vi "ExampleAll.vi"() -> ()   [LabVIEW 2009]
uses:
  C/Program Files (x86)/National Instruments/LabVIEW 2018/user.lib/ATSpectrograph/ATSpectrograph.llb/atspectrograph_portPosition_typedef.ctl
  C/Program Files (x86)/National Instruments/LabVIEW 2018/user.lib/ATSpectrograph/ATSpectrograph.llb/atspectrograph_flipper_typedef.ctl
  C/Program Files (x86)/National Instruments/LabVIEW 2018/user.lib/ATSpectrograph/ATSpectrograph.llb/atspectrograph_slitIndex_typedef.ctl
  C/Program Files (x86)/National Instruments/LabVIEW 2018/user.lib/ATSpectrograph/ATSpectrograph.llb/atspectrograph_shutterMode_typedef.ctl
panel:
  in  "Device":i32 min=0 max=1
  in  "Tab Control":T1(tab)
  in  "Grating Offset":i32
  out "SetGratingOffset":string
  in  "Detector Offset":i32
  out "SetDetectorOffset":string
  out "WavelengthReset":string
  out "SetGrating":string
  in  "Grating":i32
  in  "Turret":i32
  out "SetTurret":string
  in  "SetGratingOffset":bool
  in  "SetDetectorOffset":bool
  in  "WavelengthReset":bool
  in  "SetGrating":bool
  in  "SetTurret":bool
  out "blaze":string
  out "Grating Offset":i32
  out "Detector Offset":i32
  out "offset":i32
  out "home":i32
  out "lines/mm":sgl format="%.2f"
  out "Grating":i32
  out "No Gratings":i32
  out "Turret":i32
  out "Is Grating ?":string
  out "GetGratingOffset":string
  out "GetDetectorOffset":string
  out "GetGratingInfo":string
  out "GetGrating":string
  out "GetNumberGratings":string
  out "GetTurret":string
  out "GratingIsPresent":string
  in  "Exit Port":T2
  in  "Entrance Port":T2
  out "GetCalibration":string
  out "SetNumberPixels":string
  out "SetPixelWidth":string
  out "Max Dispersion":sgl
  out "Min Dispersion":sgl
  in  "Number Pixels":i32 caption="Numeric"
  in  "Pixel Width":sgl caption="Numeric" format="%_3g"
  out "GotoZeroOrder":string
  out "SetWavelength":string
  in  "Wavelength":sgl format="%.2f"
  in  "GoToZeroOrder":bool
  out "Max Wavelength":sgl format="%.2f"
  out "Min Wavelength":sgl format="%.2f"
  out "Is Wavelength ?":string
  out "WavelengthIsPresent":string
  out "GetWavelengthLimits":string
  out "At Zero Order ?":string
  out "AtZeroOrder":string
  out "Wavelength":sgl format="%.2f"
  in  "SetWavelength 2":bool
  out "GetWavelength":string
  out "GetPixelWidth":string
  out "GetPixelCalibrationCoefficients":string
  out "GetNumberPixels":string
  out "Pixel Width":sgl format="%.2f"
  out "Number Pixels":i32
  out "A":sgl format="%.2f"
  out "B":sgl format="%.2f"
  out "C":sgl format="%.2f"
  out "D":sgl format="%.2f"
  in  "Slit":T3
  in  "SetSlit":bool
  in  "ResetSlit":bool
  in  "Slit Width":sgl format="%.2f"
  out "SetSlit":string
  out "ResetSlit":string
  out "Is Slit present ?":string
  out "GetSlitWidth":string
  out "SlitIsPresent":string
  out "Slit width (mm)":sgl format="%.2f"
  out "GetSlitZeroPosition":string
  out "SetSlitZeroPosition":string
  in  "SlitZeroPosition":i32
  in  "SlitZeroPositionGet":bool
  in  "SlitZeroPositionSet":bool caption="SetSlitZeroPosition"
  out "x1":i32
  out "y1":i32
  out "x2":i32
  out "y2":i32
  out "GetSlitCoefficients":string
  out "Shutter":T4
  in  "Mode":T4
  in  "SetShutter":bool
  out "Is Mode Possible ?":string
  out "Is Shutter ?":string
  out "SetShutter":string
  out "IsModePossible":string
  out "GetShutter":string
  out "ShutterIsPresent":string
  out "Port":T2
  in  "Flipper Port":T2
  in  "Flipper Mirror":T5
  out "High":sgl format="%.2f"
  in  "FlipperReset":bool
  out "FlipperReset":string
  in  "SetPort":bool
  out "Low":sgl format="%.2f"
  out "Is Flipper ?":string
  out "SetPort":string
  out "GetCCDLimits":string
  out "FlipperIsPresent":string
  out "GetFlipperMirror":string
  out "SetFlipperMirrorPosition":string
  in  "SetFlipperMirrorPosition":bool
  in  "Position":i32
  out "GetFlipperMirrorPosition":string
  out "Mirror Max Position":i32
  out "Mirror Position":i32
  out "GetFlipperMirrorMaxPosition":string
  in  "ResetFocusMirror":bool
  in  "MoveFocusMirror":bool
  in  "Steps":i32
  out "FocusMirrorReset":string
  out "SetFocusMirror":string
  out "FocusMirrorIsPresent":string
  out "GetFocusMirror":string
  out "GetFocusMirrorMaxSteps":string
  out "Max Steps":i32
  out "Is Focus Mirror ?":string
  out "Focus":i32
  in  "Iris":T2
  in  "SetIris":bool
  out "SetIris":string
  in  "Value":i32
  out "Iris Value":i32
  out "Is Iris ?":string
  out "GetIris":string
  out "IrisIsPresent":string
  in  "Filter info":string caption="String"
  out "Filter Info":string
  in  "SetFilterInfo":bool
  out "SetFilterInfo":string
  in  "Filter":i32
  in  "SetFilter":bool
  out "Filter":i32
  out "Is Filter ?":string
  out "SetFilter":string
  out "GetFilterInfo":string
  out "GetFilter":string
  out "FilterIsPresent":string
  in  "ResetFilter 2":bool
  out "ResetFilter":string
  in  "Line":i32
  out "Line 2":i32
  in  "State":i32
  in  "Set Accessory":bool
  out "Line 1":i32
  out "Is Accessory ?":string
  out "SetAccessory":string
  out "GetAccessory":string
  out "AccessoryIsPresent":string
  in  "Set Params":bool
  out "Set Optical Parameters":string
  in  "Focal tilt":sgl format="%.2f"
  in  "Angular deviation":sgl format="%.2f"
  in  "Focal length":sgl format="%.4f"
  out "Initializing":bool
  in  "STOP if TRUE":bool
  out "Focal tilt":sgl format="%.2f"
  out "Angular deviation":sgl format="%.2f"
  out "Focal length":sgl format="%.4f"
  out "Serial Number":string
  out "No of devices":i32
  out "GetOpticalParameters":string
  out "GetSerialNumber":string
  out "GetNumberDevices":string
  out "Close":string
  out "Initialize":string
  # "INITIALIZATION"
  # "SDK RETURN VALUES"
  # "SHAMROCK PARAMETERS"
  # "ACTIONS"
  # "SDK RETURN VALUES"
  # "SHAMROCK PARAMETERS"
  # "ACTIONS"
  # "SDK RETURN VALUES"
  # "SHAMROCK PARAMETERS"
  # "ACTIONS"
  # "nm"
  # "Dispersion range"
  # "SDK RETURN VALUES"
  # "SHAMROCK PARAMETERS"
  # "ACTIONS"
  # "Slit Zero Position"
  # "SDK RETURN VALUES"
  # "SHAMROCK PARAMETERS"
  # "ACTIONS"
  # "SDK RETURN VALUES"
  # "SHAMROCK PARAMETERS"
  # "ACTIONS"
  # "SDK RETURN VALUES"
  # "SHAMROCK PARAMETERS"
  # "ACTIONS"
  # "SDK RETURN VALUES"
  # "SHAMROCK PARAMETERS"
  # "ACTIONS"
  # "SDK RETURN VALUES"
  # "SHAMROCK PARAMETERS"
  # "ACTIONS"
  # "SDK RETURN VALUES"
  # "SHAMROCK PARAMETERS"
  # "ACTIONS"
  # "line"
  # "to state"
  # "SDK RETURN VALUES"
  # "SHAMROCK PARAMETERS"
  # "ACTIONS"
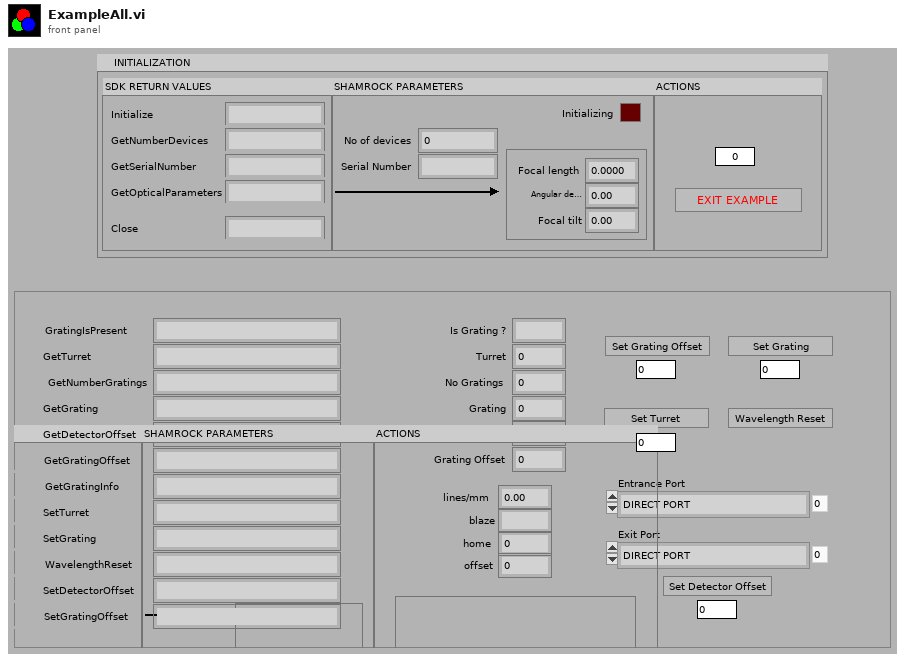
[diagram p1: front panel]
types:
  T1 = enum32{"GRATINGS", "WAVELENGTH", "SLIT", "SHUTTER", "FLIPPER MIRROR", "FOCUS MIRROR", "IRIS", "FILTER", "ACCESSORY", "OPTICALPARAMS"}
  T2 = typedef "atspectrograph_portPosition_typedef.ctl" = enum32{"DIRECT PORT", "SIDE PORT"}
  T3 = typedef "atspectrograph_slitIndex_typedef.ctl" = enum32{"Reserved (0)", "INPUT SIDE", "INPUT DIRECT", "OUTPUT SIDE", "OUTPUT DIRECT"}
  T4 = typedef "atspectrograph_shutterMode_typedef.ctl" = enum32{"CLOSED", "OPEN", "BNC"}
  T5 = typedef "atspectrograph_flipper_typedef.ctl" = enum32{"Reserved (0)", "INPUT FLIPPER", "OUTPUT FLIPPER"}
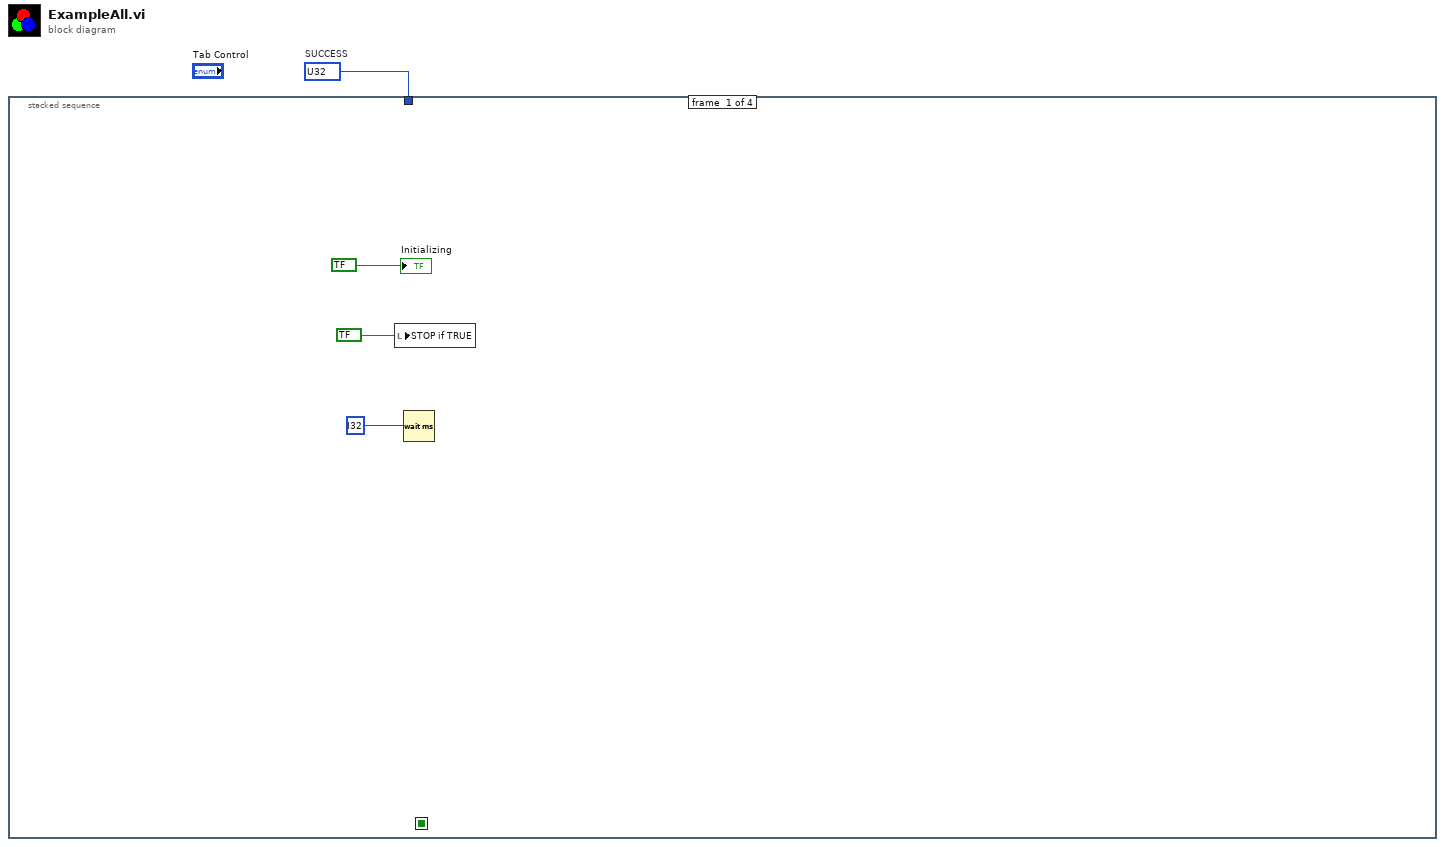
[diagram p0: block diagram]
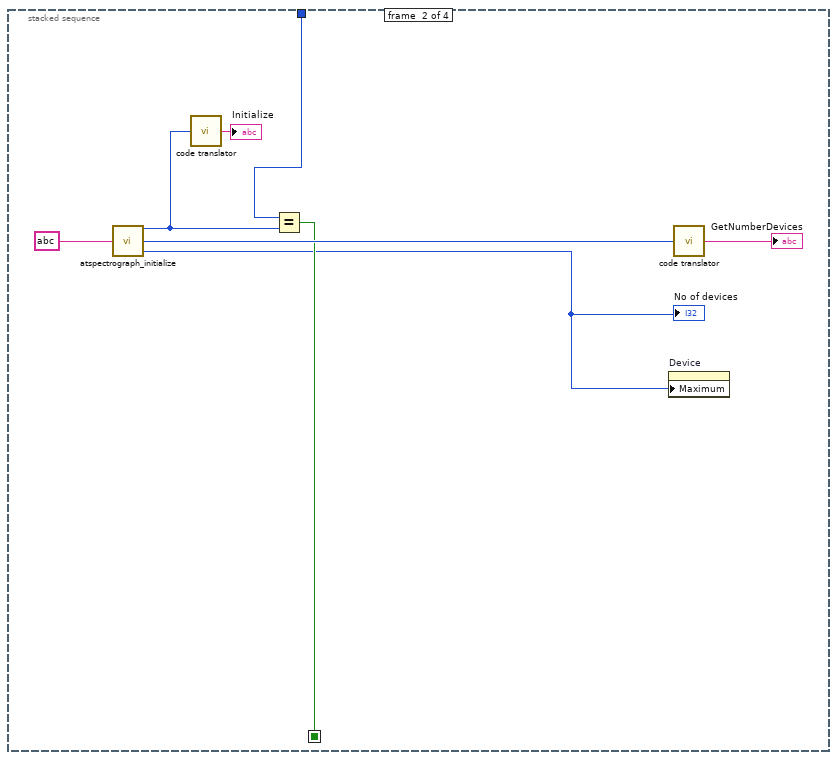
[diagram p2: hidden frame]
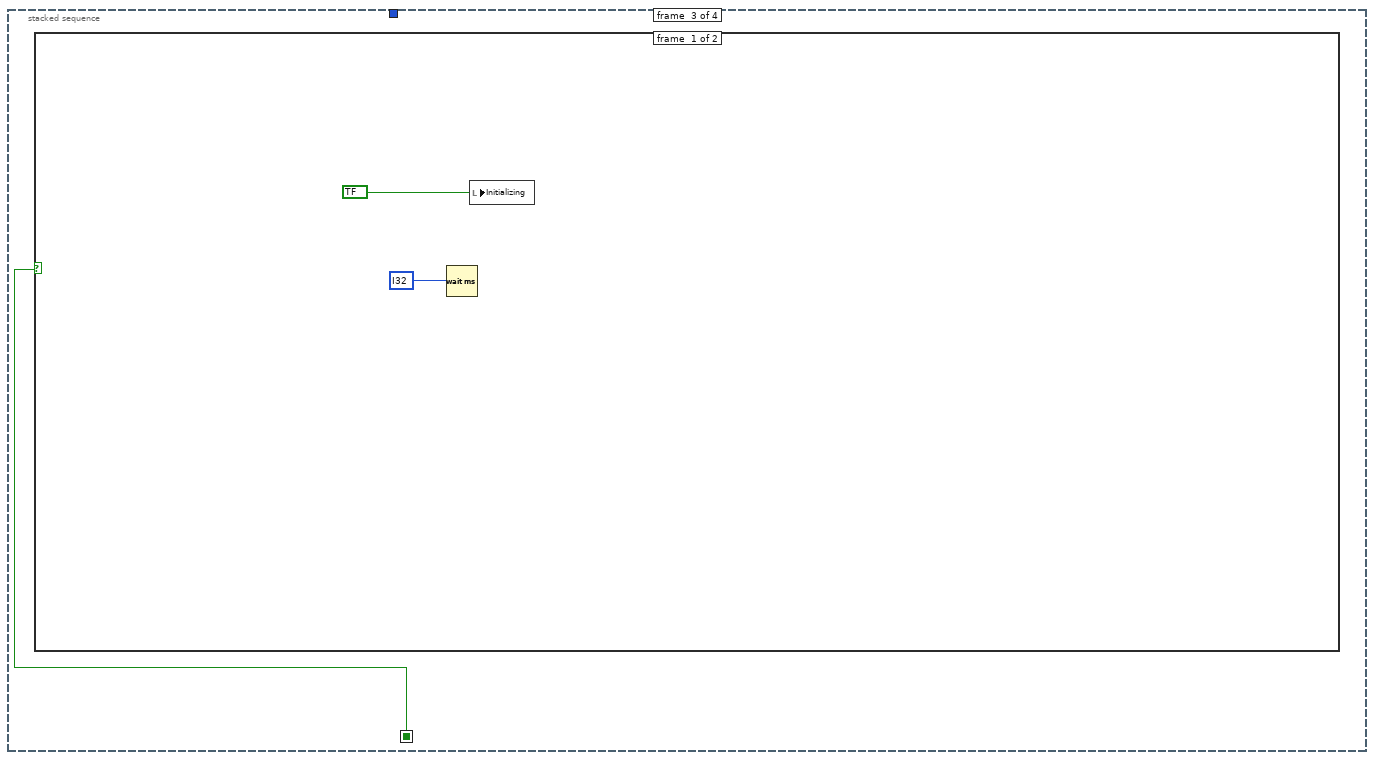
[diagram p3: hidden frame]
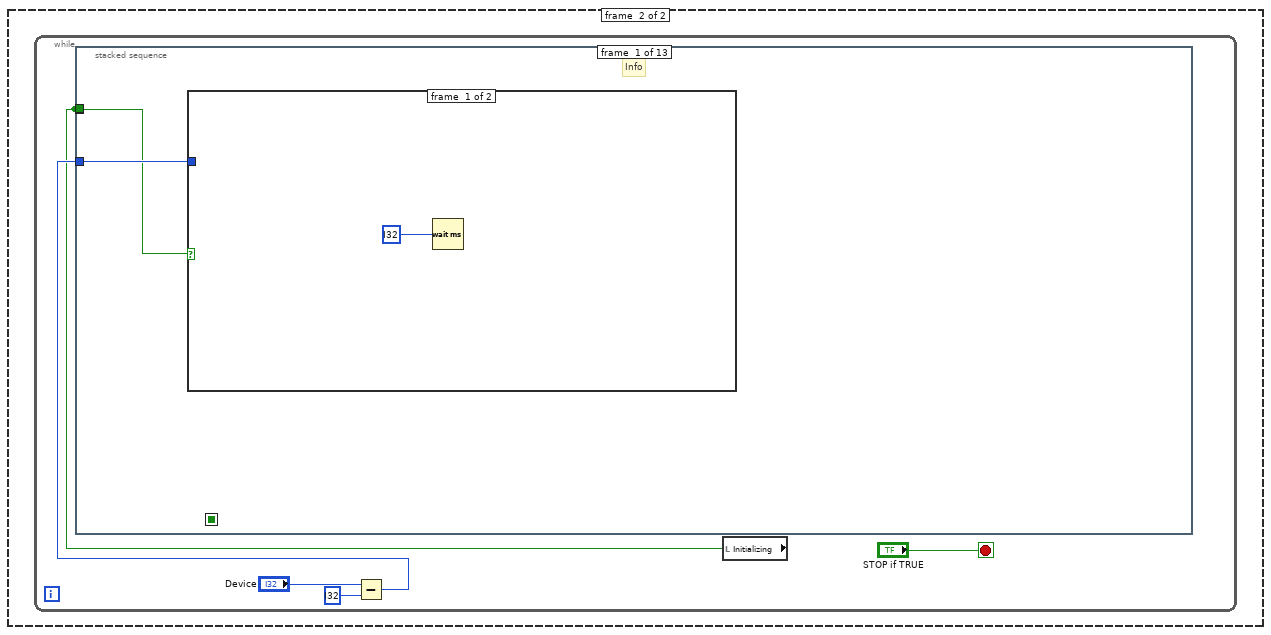
[diagram p4: hidden frame]
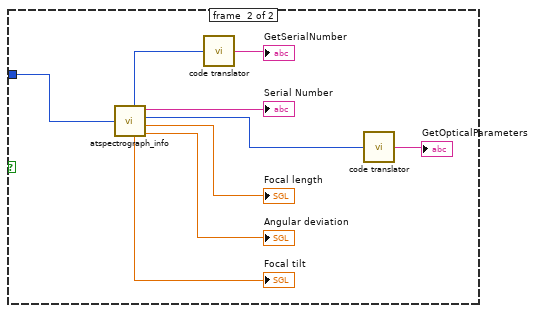
[diagram p5: hidden frame]
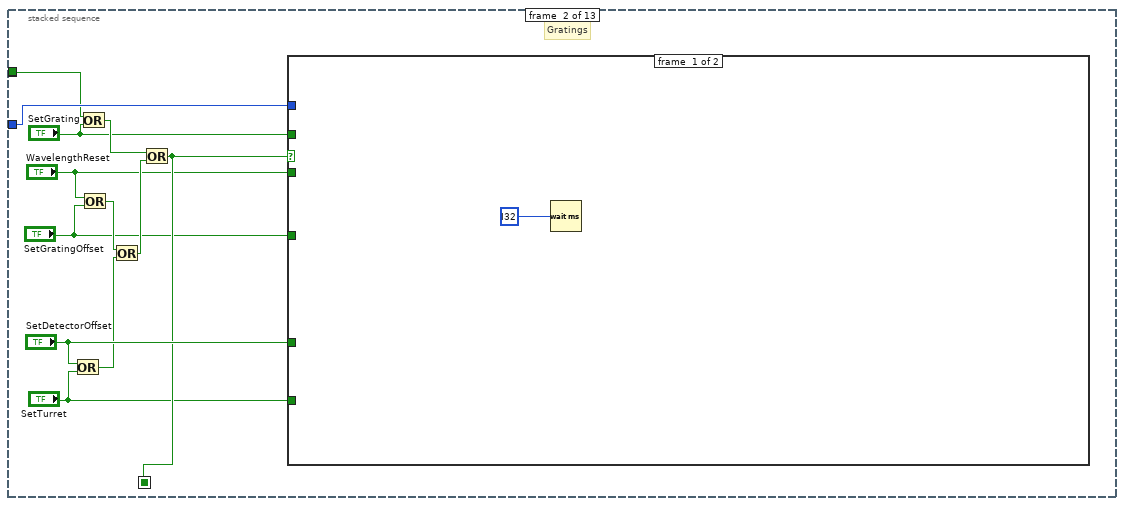
[diagram p6: hidden frame]
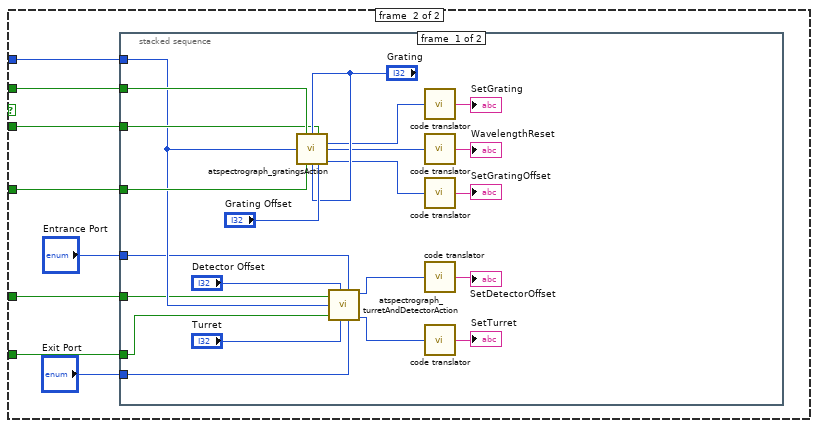
[diagram p7: hidden frame]
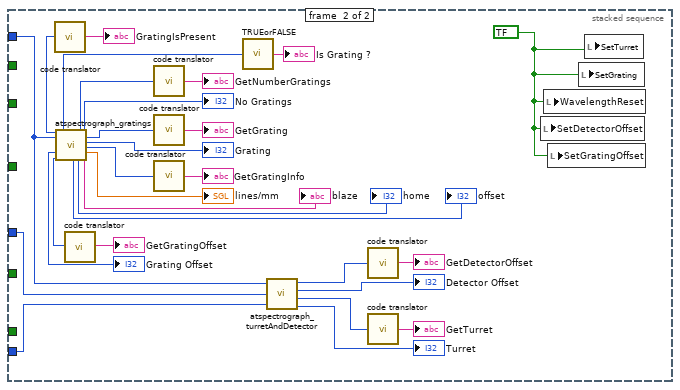
[diagram p8: hidden frame]
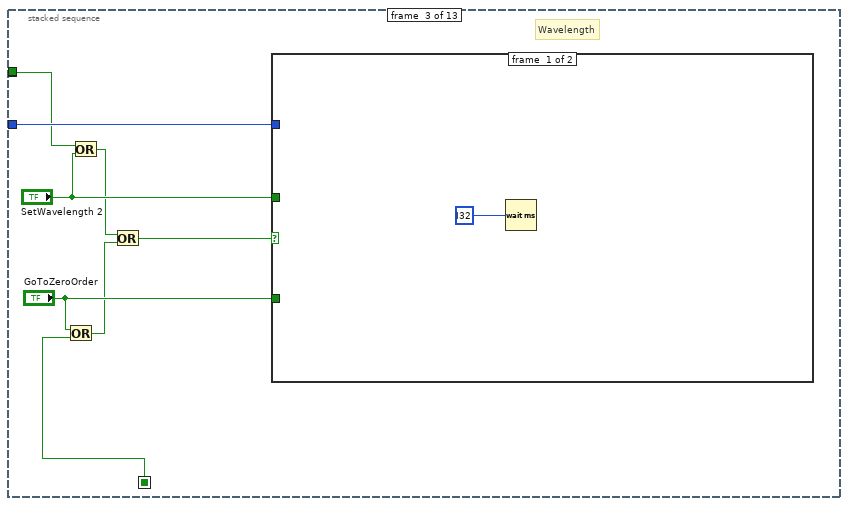
[diagram p9: hidden frame]
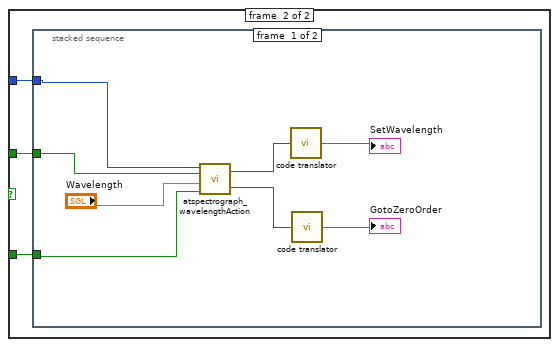
[diagram p10: hidden frame]
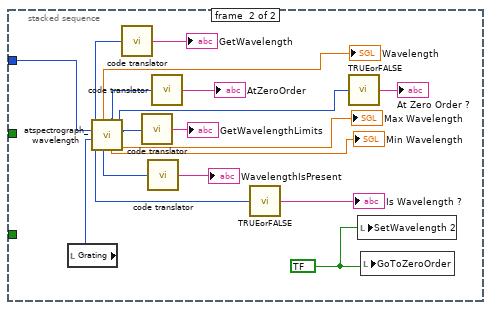
[diagram p11: hidden frame]
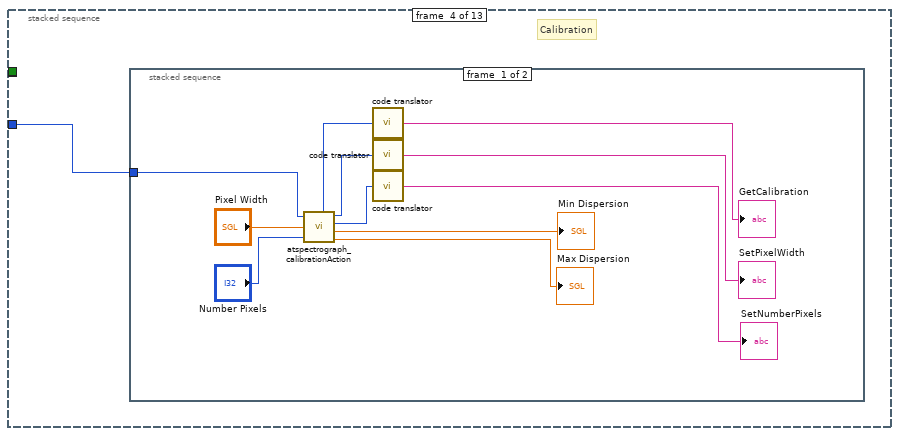
[diagram p12: hidden frame]
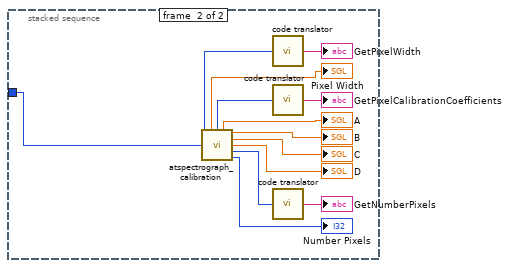
[diagram p13: hidden frame]
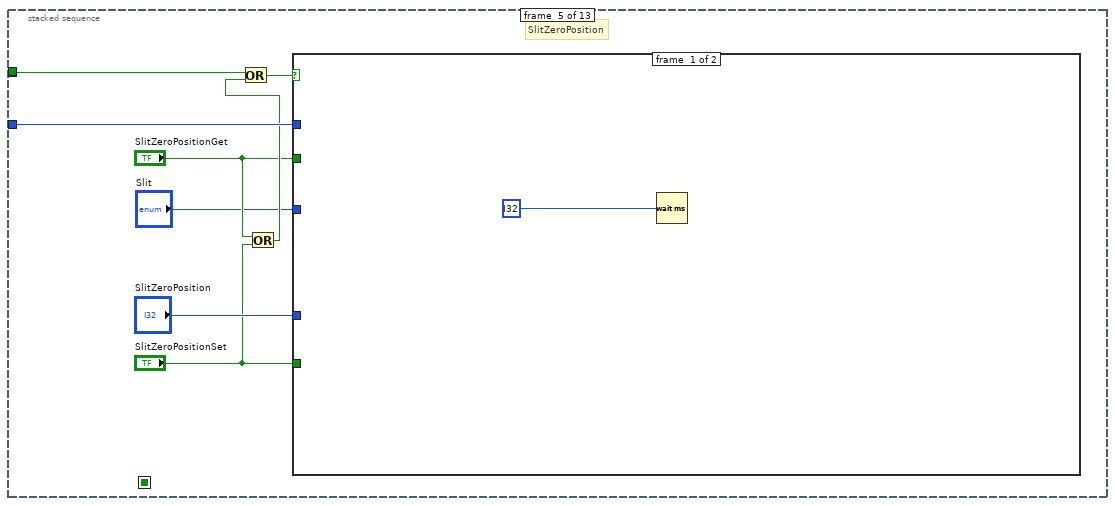
[diagram p14: hidden frame]
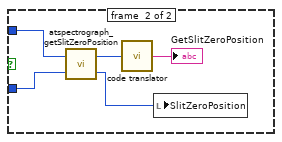
[diagram p16: hidden frame]
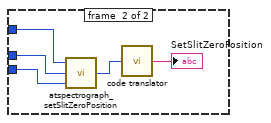
[diagram p17: hidden frame]
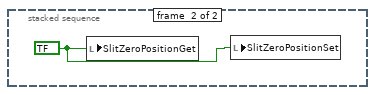
[diagram p18: hidden frame]
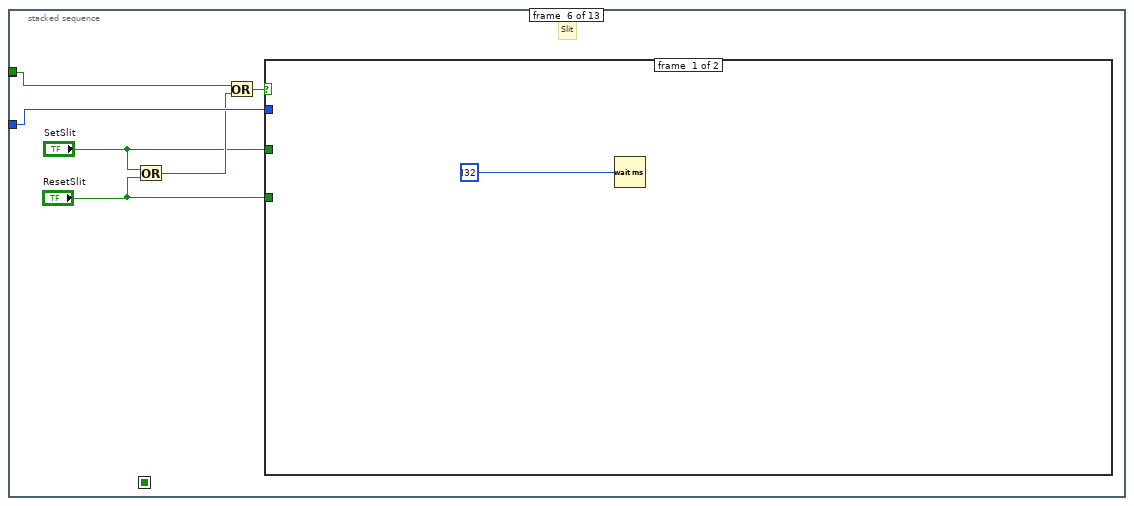
[diagram p19: hidden frame]
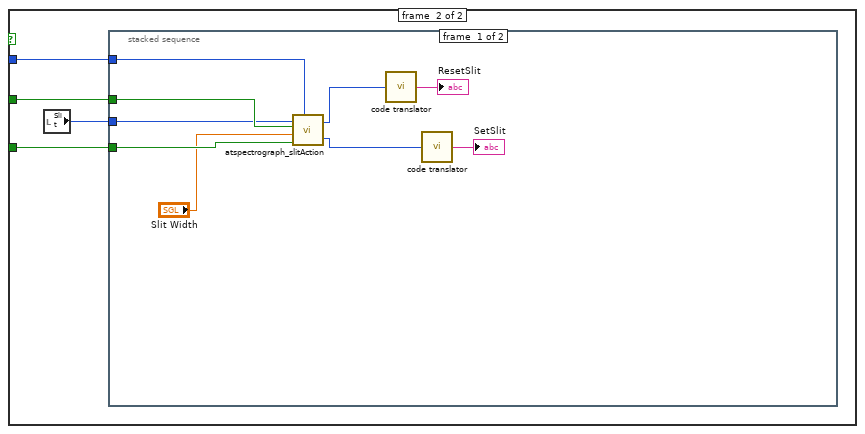
[diagram p20: hidden frame]
diagram:
  w1 = u32 ?  # SUCCESS
  n1 = stacked-sequence {
    seq-local: [_ w6 _ _] -> [_ _ w13 _]
    tunnel: w1 -> [_ w12 _ _]
    frame #0 {
      n2 = local write "STOP if TRUE"(bool ?) -> ()
      n3 = Wait (ms)(milliseconds to wait=i32 ?) -> ()  [unwired: 1 out]
      "Initializing" <- bool ?
    }
    frame #1 {
      n4 = call "atspectrograph_initialize.vi"("Initialization path"=string ?) -> ("RC_Initialize"=w9:u32, "RC_GetNumberDevices"=w8:u32, "No Devices"=w5:i32)
      "No of devices" <- w5
      n5 = call "code translator.vi"("Error code"=w9) -> ("Error description"=→"Initialize":string)
      n6 = Equal?(x=w12, y=w9) -> (x = y?=w6:bool)
      n7 = property on="Device" class="DigNum (strict)"("Maximum"=w5) -> ()  [unwired: 2 in, 2 out]
      n8 = call "code translator.vi"("Error code"=w8) -> ("Error description"=→"GetNumberDevices":string)
    }
    frame #2 {
      n9 = case shown="True" w13 {
        frame #0 {
          n10 = Wait (ms)(milliseconds to wait=i32 ?) -> ()  [unwired: 1 out]
          n11 = local write "Initializing"(bool ?) -> ()
        }
        frame #1 {
          n12 = while {
            stop <- "STOP if TRUE" stop-if-true
            n13 = Subtract(x="Device", y=i32 ?) -> (x-y=w19:i32)
            n14 = local read "Initializing"() -> (w16:bool)
            n15 = stacked-sequence {
              seq-local: [_ w37 _ _ _ _ _ _ _ _ _ _ _] -> [_ _ w111 _ _ _ _ _ _ _ _ _ _]
              tunnel: w19 -> [w22 w44 w112 w143 w175 w201 w237 w267 w312 w340 w368 w401 w425]
              tunnel: w16 -> [w21 w40 w108 _ w173 w203 w234 w262 w311 w339 w364 w398 _]
              tunnel: w16 -> [_ _ _ _ _ _ _ _ _ _ _ _ _]
              frame #0 {
                # "Info"
                n16 = case shown="True" w21 {
                  tunnel: w22 -> [_ w24]
                  frame #0 {
                    n17 = Wait (ms)(milliseconds to wait=i32 ?) -> ()  [unwired: 1 out]
                  }
                  frame #1 {
                    n18 = call "atspectrograph_info.vi"("Device No"=w24) -> ("RC_GetSerialNumber"=w28:u32, "Focal Tilt"=→"Focal tilt":sgl, "Serial Number"=→"Serial Number":string, "RC_GetOpticalParameters"=w26:u32, "Focal Length"=→"Focal length":sgl, "Angular Deviation"=→"Angular deviation":sgl)
                    n19 = call "code translator.vi"("Error code"=w28) -> ("Error description"=→"GetSerialNumber":string)
                    n20 = call "code translator.vi"("Error code"=w26) -> ("Error description"=→"GetOpticalParameters":string)
                  }
                }
              }
              frame #1 {
                # "Gratings"
                n21 = Or(x="SetDetectorOffset", y="SetTurret") -> (x .or. y?=w41:bool)
                n22 = Or(x=w40, y="SetGrating") -> (x .or. y?=w39:bool)
                n23 = Or(x="WavelengthReset", y="SetGratingOffset") -> (x .or. y?=w42:bool)
                n24 = Or(x=w42, y=w41) -> (x .or. y?=w38:bool)
                n25 = Or(x=w39, y=w38) -> (x .or. y?=w37:bool)
                n26 = case shown="True" w37 {
                  tunnel: w44 -> [_ w53]
                  tunnel: "SetDetectorOffset" -> [_ w52]
                  tunnel: "SetTurret" -> [_ w51]
                  tunnel: "WavelengthReset" -> [_ w50]
                  tunnel: "SetGratingOffset" -> [_ w49]
                  tunnel: "SetGrating" -> [_ w48]
                  frame #0 {
                    n27 = Wait (ms)(milliseconds to wait=i32 ?) -> ()  [unwired: 1 out]
                  }
                  frame #1 {
                    n28 = stacked-sequence {
                      tunnel: w48 -> [w65 _]
                      tunnel: w53 -> [w62 w78]
                      tunnel: w50 -> [w64 _]
                      tunnel: w49 -> [w63 _]
                      tunnel: w52 -> [w58 _]
                      tunnel: w51 -> [w59 _]
                      tunnel: "Entrance Port" -> [w55 w77]
                      tunnel: "Exit Port" -> [w54 w76]
                      frame #0 {
                        n29 = call "atspectrograph_gratingsAction.vi"("WavelengthReset"=w64, "Grating Offset"="Grating Offset", 7:"Grating"="Grating", 8:"Grating"="Grating", "SetGrating"=w65, "SetGratingOffset"=w63, "Device No"=w62) -> ("RC_SetGrating"=w72:u32, "RC_WavelengthReset"=w69:u32, "RC_SetGratingOffset"=w67:u32)  [unwired: 6 in]
                        n30 = call "atspectrograph_turretAndDetectorAction.vi"("SetDetectorOffset"=w58, "Detector Offset"="Detector Offset", "Device No"=w62, "SetTurret"=w59, "Turret"="Turret", "Entrance Port"=w55, "Exit Port"=w54) -> ("RC_SetDetectorOffset"=w57:u32, "RC_SetTurret"=w56:u32)  [unwired: 2 in]
                        n31 = call "code translator.vi"("Error code"=w72) -> ("Error description"=→"SetGrating":string)
                        n32 = call "code translator.vi"("Error code"=w69) -> ("Error description"=→"WavelengthReset":string)
                        n33 = call "code translator.vi"("Error code"=w67) -> ("Error description"=→"SetGratingOffset":string)
                        n34 = call "code translator.vi"("Error code"=w57) -> ("Error description"=→"SetDetectorOffset":string)
                        n35 = call "code translator.vi"("Error code"=w56) -> ("Error description"=→"SetTurret":string)
                      }
                      frame #1 {
                        w104 = bool ?
                        n36 = call "atspectrograph_gratings.vi"("Device No"=w78) -> ("No Gratings"=→"No Gratings":i32, "RC_GetNumberGratings"=w93:u32, "Is Present"=w84:i32, "RC_GratingIsPresent"=w96:u32, "RC_GetGrating"=w91:u32, "Grating"=→"Grating":i32, "RC_GetGratingInfo"=w89:u32, "Lines/mm"=→"lines/mm":sgl, "Grating Offset"=→"Grating Offset":i32, "Blaze"=→"blaze":string, "Home"=→"home":i32, "Offset"=→"offset":i32, "RC_GetGratingOffset"=w86:u32)  [unwired: 6 in]
                        n37 = call "code translator.vi"("Error code"=w96) -> ("Error description"=→"GratingIsPresent":string)
                        n38 = call "code translator.vi"("Error code"=w86) -> ("Error description"=→"GetGratingOffset":string)
                        n39 = call "code translator.vi"("Error code"=w93) -> ("Error description"=→"GetNumberGratings":string)
                        n40 = call "code translator.vi"("Error code"=w91) -> ("Error description"=→"GetGrating":string)
                        n41 = call "code translator.vi"("Error code"=w89) -> ("Error description"=→"GetGratingInfo":string)
                        n42 = call "TRUEorFALSE.vi"("bool number"=w84) -> ("String"=→"Is Grating ?":string)
                        n43 = call "atspectrograph_turretAndDetector.vi"("Device No"=w78, "Entrance Port"=w77, "Exit Port"=w76) -> ("RC_GetDetectorOffset"=w82:u32, "Detector Offset"=→"Detector Offset":i32, "RC_GetTurret"=w80:u32, "Turret"=→"Turret":i32)
                        n44 = call "code translator.vi"("Error code"=w82) -> ("Error description"=→"GetDetectorOffset":string)
                        n45 = call "code translator.vi"("Error code"=w80) -> ("Error description"=→"GetTurret":string)
                        n46 = local write "SetDetectorOffset"(w104) -> ()
                        n47 = local write "WavelengthReset"(w104) -> ()
                        n48 = local write "SetGratingOffset"(w104) -> ()
                        n49 = local write "SetGrating"(w104) -> ()
                        n50 = local write "SetTurret"(w104) -> ()
                      }
                    }
                  }
                }
              }
              frame #2 {
                # "Wavelength"
                n51 = Or(x="GoToZeroOrder", y=w111) -> (x .or. y?=w106:bool)
                n52 = Or(x=w108, y="SetWavelength 2") -> (x .or. y?=w107:bool)
                n53 = Or(x=w107, y=w106) -> (x .or. y?=w105:bool)
                n54 = case shown="True" w105 {
                  tunnel: "SetWavelength 2" -> [_ w116]
                  tunnel: "GoToZeroOrder" -> [_ w115]
                  tunnel: w112 -> [_ w114]
                  frame #0 {
                    n55 = Wait (ms)(milliseconds to wait=i32 ?) -> ()  [unwired: 1 out]
                  }
                  frame #1 {
                    n56 = stacked-sequence {
                      tunnel: w116 -> [w122 _]
                      tunnel: w115 -> [w123 _]
                      tunnel: w114 -> [w121 w137]
                      frame #0 {
                        n57 = call "atspectrograph_wavelengthAction.vi"("GoToZeroOrder"=w123, "Wavelength"="Wavelength", "SetWavelength"=w122, "Device No"=w121) -> ("RC_GotoZeroOrder"=w118:u32, "RC_SetWavelength"=w120:u32)
                        n58 = call "code translator.vi"("Error code"=w120) -> ("Error description"=→"SetWavelength":string)
                        n59 = call "code translator.vi"("Error code"=w118) -> ("Error description"=→"GotoZeroOrder":string)
                      }
                      frame #1 {
                        w142 = bool ?
                        n60 = local read "Grating"() -> (w138:i32)
                        n61 = call "atspectrograph_wavelength.vi"("Grating No"=w138, "Device No"=w137) -> ("Is Present"=w126:i32, "RC_WavelengthIsPresent"=w130:u32, "Min Wavelength"=→"Min Wavelength":sgl, "Max Wavelength"=→"Max Wavelength":sgl, "RC_GetWavelengthLimits"=w132:u32, "RC_GetWavelength"=w136:u32, "Wavelength"=→"Wavelength":sgl, "RC_AtZeroOrder"=w134:u32, "At Zero Order"=w128:i32)
                        n62 = call "code translator.vi"("Error code"=w136) -> ("Error description"=→"GetWavelength":string)
                        n63 = call "code translator.vi"("Error code"=w132) -> ("Error description"=→"GetWavelengthLimits":string)
                        n64 = call "code translator.vi"("Error code"=w130) -> ("Error description"=→"WavelengthIsPresent":string)
                        n65 = call "code translator.vi"("Error code"=w134) -> ("Error description"=→"AtZeroOrder":string)
                        n66 = call "TRUEorFALSE.vi"("bool number"=w126) -> ("String"=→"Is Wavelength ?":string)
                        n67 = call "TRUEorFALSE.vi"("bool number"=w128) -> ("String"=→"At Zero Order ?":string)
                        n68 = local write "SetWavelength 2"(w142) -> ()
                        n69 = local write "GoToZeroOrder"(w142) -> ()
                      }
                    }
                  }
                }
              }
              frame #3 {
                # "Calibration"
                n70 = stacked-sequence {
                  tunnel: w143 -> [w145 w164]
                  frame #0 {
                    n71 = call "atspectrograph_calibrationAction.vi"("Device No"=w145, "Set Pixel Width"="Pixel Width", "Set Number Pixels"="Number Pixels") -> ("RC_SetPixelWidth"=w152:u32, "RC_SetNumberPixels"=w150:u32, "Wavelength First Pixel"=→"Min Dispersion":sgl, "Wavelength Last Pixel"=→"Max Dispersion":sgl, "RC_GetCalibration"=w154:u32)
                    n72 = call "code translator.vi"("Error code"=w154) -> ("Error description"=→"GetCalibration":string)
                    n73 = call "code translator.vi"("Error code"=w152) -> ("Error description"=→"SetPixelWidth":string)
                    n74 = call "code translator.vi"("Error code"=w150) -> ("Error description"=→"SetNumberPixels":string)
                  }
                  frame #1 {
                    n75 = call "atspectrograph_calibration.vi"("Device No"=w164) -> ("B"=→"B":sgl, "C"=→"C":sgl, "D"=→"D":sgl, "RC_GetNumberPixels"=w156:u32, "Number Pixels"=→"Number Pixels":i32, "A"=→"A":sgl, "RC_GetPixelCalibrationCoefficients"=w161:u32, "Width"=→"Pixel Width":sgl, "RC_GetPixelWidth"=w163:u32)  [unwired: 2 in, 4 out]
                    n76 = call "code translator.vi"("Error code"=w163) -> ("Error description"=→"GetPixelWidth":string)
                    n77 = call "code translator.vi"("Error code"=w161) -> ("Error description"=→"GetPixelCalibrationCoefficients":string)
                    n78 = call "code translator.vi"("Error code"=w156) -> ("Error description"=→"GetNumberPixels":string)
                  }
                }
              }
              frame #4 {
                # "SlitZeroPosition"
                n79 = Or(x="SlitZeroPositionGet", y="SlitZeroPositionSet") -> (x .or. y?=w170:bool)
                n80 = Or(x=w173, y=w170) -> (x .or. y?=w174:bool)
                n81 = case shown="True" w174 {
                  tunnel: w175 -> [_ w181]
                  tunnel: "SlitZeroPositionGet" -> [_ w180]
                  tunnel: "SlitZeroPositionSet" -> [_ w179]
                  tunnel: "Slit" -> [_ w178]
                  tunnel: "SlitZeroPosition" -> [_ w177]
                  frame #0 {
                    n82 = Wait (ms)(milliseconds to wait=i32 ?) -> ()  [unwired: 1 out]
                  }
                  frame #1 {
                    n83 = stacked-sequence {
                      tunnel: w181 -> [w185 _]
                      tunnel: w180 -> [w186 _]
                      tunnel: w179 -> [w184 _]
                      tunnel: w178 -> [w183 _]
                      tunnel: w177 -> [w182 _]
                      frame #0 {
                        n84 = case shown="True" w186 {
                          tunnel: w185 -> [_ w191]
                          tunnel: w183 -> [_ w187]
                          frame #0 {
                          }
                          frame #1 {
                            n85 = call "atspectrograph_getSlitZeroPosition.vi"("Slit Index"=w187, "Device No"=w191) -> ("Slit Zero Position (mm)"=w188:i32, "RC_GetSlitZeroPosition"=w190:u32)
                            n86 = call "code translator.vi"("Error code"=w190) -> ("Error description"=→"GetSlitZeroPosition":string)
                            n87 = local write "SlitZeroPosition"(w188) -> ()
                          }
                        }
                        n88 = case shown="True" w184 {
                          tunnel: w185 -> [_ w196]
                          tunnel: w183 -> [_ w193]
                          tunnel: w182 -> [_ w192]
                          frame #0 {
                          }
                          frame #1 {
                            n89 = call "atspectrograph_setSlitZeroPosition.vi"("Offset"=w192, "Slit Index"=w193, "Device No"=w196) -> ("RC_SetSlitZeroPosition"=w195:u32)
                            n90 = call "code translator.vi"("Error code"=w195) -> ("Error description"=→"SetSlitZeroPosition":string)
                          }
                        }
                      }
                      frame #1 {
                        w197 = bool ?
                        n91 = local write "SlitZeroPositionGet"(w197) -> ()
                        n92 = local write "SlitZeroPositionSet"(w197) -> ()
                      }
                    }
                  }
                }
              }
              frame #5 {
                # "Slit"
                n93 = Or(x="SetSlit", y="ResetSlit") -> (x .or. y?=w200:bool)
                n94 = Or(x=w203, y=w200) -> (x .or. y?=w202:bool)
                n95 = case shown="True" w202 {
                  tunnel: w201 -> [_ w208]
                  tunnel: "SetSlit" -> [_ w207]
                  tunnel: "ResetSlit" -> [_ w206]
                  frame #0 {
                    n96 = Wait (ms)(milliseconds to wait=i32 ?) -> ()  [unwired: 1 out]
                  }
                  frame #1 {
                    n97 = local read "Slit"() -> (w205:T3)
                    n98 = stacked-sequence {
                      tunnel: w208 -> [w217 w225]
                      tunnel: w207 -> [w216 _]
                      tunnel: w206 -> [w215 _]
                      tunnel: w205 -> [w214 w233]
                      frame #0 {
                        n99 = call "atspectrograph_slitAction.vi"("Slit"=w214, "Set Slit"=w216, "Slit Width"="Slit Width", "Reset Slit"=w215, "Device No"=w217) -> ("RC_ResetSlit"=w209:u32, "RC_SetSlit"=w211:u32)
                        n100 = call "code translator.vi"("Error code"=w209) -> ("Error description"=→"ResetSlit":string)
                        n101 = call "code translator.vi"("Error code"=w211) -> ("Error description"=→"SetSlit":string)
                      }
                      frame #1 {
                        w218 = bool ?
                        n102 = call "atspectrograph_slit.vi"("Device No"=w225, "Slit Index"=w233) -> ("RC_SlitIsPresent"=w226:u32, "RC_GetSlitWidth"=w227:u32, "Is Present"=w228:i32, "Slit Width (mm)"=→"Slit width (mm)":sgl)
                        n103 = call "atspectrograph_getSlitCoefficients.vi"("Device No"=w225) -> ("y2"=→"y2":i32, "x2"=→"x2":i32, "y1"=→"y1":i32, "x1"=→"x1":i32, "RC_GetSlitCoefficients"=w223:u32)
                        n104 = call "code translator.vi"("Error code"=w226) -> ("Error description"=→"SlitIsPresent":string)
                        n105 = call "code translator.vi"("Error code"=w227) -> ("Error description"=→"GetSlitWidth":string)
                        n106 = call "TRUEorFALSE.vi"("bool number"=w228) -> ("String"=→"Is Slit present ?":string)
                        n107 = call "code translator.vi"("Error code"=w223) -> ("Error description"=→"GetSlitCoefficients":string)
                        n108 = local write "ResetSlit"(w218) -> ()
                        n109 = local write "SetSlit"(w218) -> ()
                      }
                    }
                  }
                }
              }
              frame #6 {
                # "Shutter"
                n110 = Or(x=w234, y="SetShutter") -> (x .or. y?=w235:bool)
                n111 = case shown="True" w235 {
                  tunnel: w237 -> [_ w240]
                  tunnel: "SetShutter" -> [_ w239]
                  frame #0 {
                    n112 = Wait (ms)(milliseconds to wait=i32 ?) -> ()  [unwired: 1 out]
                  }
                  frame #1 {
                    n113 = stacked-sequence {
                      seq-local: ["Mode" _] -> [_ w257]
                      tunnel: w240 -> [w244 w258]
                      tunnel: w239 -> [w245 _]
                      frame #0 {
                        n114 = call "atspectrograph_shutterAction.vi"("Mode"="Mode", "SetShutter"=w245, "Device No"=w244) -> ("RC_SetShutter"=w243:u32)
                        n115 = call "code translator.vi"("Error code"=w243) -> ("Error description"=→"SetShutter":string)
                      }
                      frame #1 {
                        n116 = call "atspectrograph_shutter.vi"("Device No"=w258, "Mode"=w257) -> ("RC_ShutterIsPresent"=w256:u32, "Is Mode Possible"=w248:i32, "Is Present"=w249:i32, "RC_GetShutter"=w254:u32, "Shutter"=→"Shutter":T4, "RC_IsModePossible"=w252:u32)
                        n117 = call "code translator.vi"("Error code"=w256) -> ("Error description"=→"ShutterIsPresent":string)
                        n118 = call "code translator.vi"("Error code"=w252) -> ("Error description"=→"IsModePossible":string)
                        n119 = call "code translator.vi"("Error code"=w254) -> ("Error description"=→"GetShutter":string)
                        n120 = call "TRUEorFALSE.vi"("bool number"=w248) -> ("String"=→"Is Mode Possible ?":string)
                        n121 = call "TRUEorFALSE.vi"("bool number"=w249) -> ("String"=→"Is Shutter ?":string)
                        n122 = local write "SetShutter"(bool ?) -> ()
                      }
                    }
                  }
                }
              }
              frame #7 {
                # "Flipper Mirror"
                n123 = Or(x=w262, y="SetFlipperMirrorPosition") -> (x .or. y?=w261:bool)
                n124 = Or(x="SetPort", y="FlipperReset") -> (x .or. y?=w264:bool)
                n125 = Or(x=w261, y=w264) -> (x .or. y?=w263:bool)
                n126 = case shown="True" w263 {
                  tunnel: "SetPort" -> [_ w273]
                  tunnel: "FlipperReset" -> [_ w272]
                  tunnel: w267 -> [_ w271]
                  tunnel: "SetFlipperMirrorPosition" -> [_ w269]
                  frame #0 {
                    n127 = Wait (ms)(milliseconds to wait=i32 ?) -> ()  [unwired: 1 out]
                  }
                  frame #1 {
                    n128 = stacked-sequence {
                      tunnel: w273 -> [w282 _]
                      tunnel: w272 -> [w281 _]
                      tunnel: w271 -> [w284 w294]
                      tunnel: "Flipper Mirror" -> [w283 w295]
                      tunnel: w269 -> [w278 _]
                      frame #0 {
                        n129 = call "atspectrograph_flipperMirrorAction.vi"("Device No"=w284, "Position"="Position", "SetFlipperMirrorPosition"=w278, "FlipperReset"=w281, 8:"Flipper Port", "SetPort"=w282, 10:w283) -> ("RC_SetFlipperMirrorPosition"=w276:u32, "RC_FlipperReset"=w280:u32, "RC_SetPort"=w279:u32)  [unwired: 1 in]
                        n130 = call "code translator.vi"("Error code"=w279) -> ("Error description"=→"SetPort":string)
                        n131 = call "code translator.vi"("Error code"=w280) -> ("Error description"=→"FlipperReset":string)
                        n132 = call "code translator.vi"("Error code"=w276) -> ("Error description"=→"SetFlipperMirrorPosition":string)
                      }
                      frame #1 {
                        w296 = bool ?
                        n133 = call "atspectrograph_flipperMirror.vi"("Flipper"=w295, "Device No"=w294) -> ("High"=→"High":sgl, "RC_GetCCDLimits"=w301:u32, "Low"=→"Low":sgl, "Flipper Port"=→"Port":T2, "RC_GetFlipperMirror"=w298:u32, "Is Present"=w297:i32, "RC_FlipperIsPresent"=w300:u32)
                        n134 = call "atspectrograph_flipperMirrorPosition.vi"("Device No"=w294, "Flipper"=w295) -> ("RC_GetFlipperMirrorPosition"=w291:u32, "Position"=→"Mirror Position":i32, "RC_GetFlipperMirrorMaxPosition"=w289:u32, "Max Position"=→"Mirror Max Position":i32)
                        n135 = call "code translator.vi"("Error code"=w298) -> ("Error description"=→"GetFlipperMirror":string)
                        n136 = call "code translator.vi"("Error code"=w301) -> ("Error description"=→"GetCCDLimits":string)
                        n137 = call "code translator.vi"("Error code"=w300) -> ("Error description"=→"FlipperIsPresent":string)
                        n138 = call "code translator.vi"("Error code"=w291) -> ("Error description"=→"GetFlipperMirrorPosition":string)
                        n139 = call "code translator.vi"("Error code"=w289) -> ("Error description"=→"GetFlipperMirrorMaxPosition":string)
                        n140 = call "TRUEorFALSE.vi"("bool number"=w297) -> ("String"=→"Is Flipper ?":string)
                        n141 = local write "SetFlipperMirrorPosition"(w296) -> ()
                        n142 = local write "SetPort"(w296) -> ()
                        n143 = local write "FlipperReset"(w296) -> ()
                      }
                    }
                  }
                }
              }
              frame #8 {
                # "Focus Mirror"
                n144 = Or(x="ResetFocusMirror", y="MoveFocusMirror") -> (x .or. y?=w310:bool)
                n145 = Or(x=w311, y=w310) -> (x .or. y?=w309:bool)
                n146 = case shown="True" w309 {
                  tunnel: w312 -> [_ w316]
                  tunnel: "ResetFocusMirror" -> [_ w315]
                  tunnel: "MoveFocusMirror" -> [_ w314]
                  frame #0 {
                    n147 = Wait (ms)(milliseconds to wait=i32 ?) -> ()  [unwired: 1 out]
                  }
                  frame #1 {
                    n148 = stacked-sequence {
                      tunnel: w316 -> [w324 w336]
                      tunnel: w315 -> [w323 _]
                      tunnel: w314 -> [w322 _]
                      frame #0 {
                        n149 = call "atspectrograph_focusMirrorAction.vi"("focus"="Steps", "SetFocusMirror"=w322, "FocusMirrorReset"=w323, "Device No"=w324) -> ("RC_SetFocusMirror"=w318:u32, "RC_FocusMirrorReset"=w317:u32)
                        n150 = call "code translator.vi"("Error code"=w317) -> ("Error description"=→"FocusMirrorReset":string)
                        n151 = call "code translator.vi"("Error code"=w318) -> ("Error description"=→"SetFocusMirror":string)
                      }
                      frame #1 {
                        w325 = bool ?
                        n152 = call "atspectrograph_focusMirror.vi"("Device No"=w336) -> ("RC_FocusMirrorIsPresent"=w332:u32, "Max Steps"=→"Max Steps":i32, "Is Present"=w328:i32, "RC_GetFocusMirror"=w331:u32, "Focus"=→"Focus":i32, "RC_GetFocusMirrorMaxSteps"=w330:u32)
                        n153 = call "TRUEorFALSE.vi"("bool number"=w328) -> ("String"=→"Is Focus Mirror ?":string)
                        n154 = call "code translator.vi"("Error code"=w332) -> ("Error description"=→"FocusMirrorIsPresent":string)
                        n155 = call "code translator.vi"("Error code"=w331) -> ("Error description"=→"GetFocusMirror":string)
                        n156 = call "code translator.vi"("Error code"=w330) -> ("Error description"=→"GetFocusMirrorMaxSteps":string)
                        n157 = local write "ResetFocusMirror"(w325) -> ()
                        n158 = local write "MoveFocusMirror"(w325) -> ()
                      }
                    }
                  }
                }
              }
              frame #9 {
                # "Iris"
                n159 = Or(x=w339, y="SetIris") -> (x .or. y?=w338:bool)
                n160 = case shown="True" w338 {
                  tunnel: w340 -> [_ w344]
                  tunnel: "SetIris" -> [_ w343]
                  frame #0 {
                    n161 = Wait (ms)(milliseconds to wait=i32 ?) -> ()  [unwired: 1 out]
                  }
                  frame #1 {
                    n162 = stacked-sequence {
                      tunnel: w344 -> [w350 w360]
                      tunnel: w343 -> [w349 _]
                      tunnel: "Iris" -> [w345 w352]
                      frame #0 {
                        n163 = call "atspectrograph_irisAction.vi"("Port"=w345, "Value"="Value", "SetIris"=w349, "Device No"=w350) -> ("RC_SetIris"=w346:u32)
                        n164 = call "code translator.vi"("Error code"=w346) -> ("Error description"=→"SetIris":string)
                      }
                      frame #1 {
                        n165 = call "atspectrograph_iris.vi"("Device No"=w360, "Iris"=w352) -> ("RC_IrisIsPresent"=w357:u32, "Is Present"=w354:i32, "RC_GetIris"=w356:u32, "Iris Value"=→"Iris Value":i32)
                        n166 = call "TRUEorFALSE.vi"("bool number"=w354) -> ("String"=→"Is Iris ?":string)
                        n167 = call "code translator.vi"("Error code"=w357) -> ("Error description"=→"IrisIsPresent":string)
                        n168 = call "code translator.vi"("Error code"=w356) -> ("Error description"=→"GetIris":string)
                        n169 = local write "SetIris"(bool ?) -> ()
                      }
                    }
                  }
                }
              }
              frame #10 {
                # "Filter"
                n170 = Or(x="SetFilter", y="SetFilterInfo") -> (x .or. y?=w365:bool)
                n171 = Or(x=w364, y="ResetFilter 2") -> (x .or. y?=w363:bool)
                n172 = Or(x=w363, y=w365) -> (x .or. y?=w361:bool)
                n173 = case shown="True" w361 {
                  tunnel: w368 -> [_ w373]
                  tunnel: "SetFilter" -> [_ w372]
                  tunnel: "SetFilterInfo" -> [_ w371]
                  tunnel: "ResetFilter 2" -> [_ w370]
                  frame #0 {
                    n174 = Wait (ms)(milliseconds to wait=i32 ?) -> ()  [unwired: 1 out]
                  }
                  frame #1 {
                    n175 = stacked-sequence {
                      tunnel: w373 -> [w382 w395]
                      tunnel: w372 -> [w385 _]
                      tunnel: w371 -> [w384 _]
                      tunnel: w370 -> [w376 _]
                      frame #0 {
                        n176 = call "atspectrograph_filterAction.vi"("Device No"=w382, "Filter info"="Filter info", "FilterReset"=w376, 7:"Filter"="Filter", "SetFilterInfo"=w384, 9:"Filter"="Filter", "SetFilter"=w385) -> ("RC_SetFilterInfo"=w377:u32, "RC_SetFilter"=w378:u32, "RC_FilterReset"=w374:u32)  [unwired: 1 in]
                        n177 = call "code translator.vi"("Error code"=w378) -> ("Error description"=→"SetFilter":string)
                        n178 = call "code translator.vi"("Error code"=w374) -> ("Error description"=→"ResetFilter":string)
                        n179 = call "code translator.vi"("Error code"=w377) -> ("Error description"=→"SetFilterInfo":string)
                      }
                      frame #1 {
                        w387 = bool ?
                        n180 = call "atspectrograph_filter.vi"("Device No"=w395) -> ("RC_FilterIsPresent"=w394:u32, "Filter Info"=→"Filter Info":string, "Is Present"=w388:i32, "RC_GetFilter"=w386:u32, "Filter"=→"Filter":i32, "RC_GetFilterInfo"=w391:u32)
                        n181 = call "code translator.vi"("Error code"=w394) -> ("Error description"=→"FilterIsPresent":string)
                        n182 = call "code translator.vi"("Error code"=w391) -> ("Error description"=→"GetFilterInfo":string)
                        n183 = call "code translator.vi"("Error code"=w386) -> ("Error description"=→"GetFilter":string)
                        n184 = call "TRUEorFALSE.vi"("bool number"=w388) -> ("String"=→"Is Filter ?":string)
                        n185 = local write "ResetFilter 2"(w387) -> ()
                        n186 = local write "SetFilter"(w387) -> ()
                        n187 = local write "SetFilterInfo"(w387) -> ()
                      }
                    }
                  }
                }
              }
              frame #11 {
                # "Accessory"
                n188 = Or(x=w398, y="Set Accessory") -> (x .or. y?=w400:bool)
                n189 = case shown="True" w400 {
                  tunnel: w401 -> [_ w404]
                  tunnel: "Set Accessory" -> [_ w403]
                  frame #0 {
                    n190 = Wait (ms)(milliseconds to wait=i32 ?) -> ()  [unwired: 1 out]
                  }
                  frame #1 {
                    n191 = stacked-sequence {
                      tunnel: w404 -> [w407 w417]
                      tunnel: w403 -> [w410 _]
                      frame #0 {
                        n192 = call "atspectrograph_accessoryAction.vi"("State"="State", "Line"="Line", "Set Accessory"=w410, "Device No"=w407) -> ("RC_SetAccessory"=w406:u32)
                        n193 = call "code translator.vi"("Error code"=w406) -> ("Error description"=→"SetAccessory":string)
                      }
                      frame #1 {
                        n194 = call "atspectrograph_accessory.vi"("Device No"=w417) -> ("Line 2"=→"Line 2":i32, "Line 1"=→"Line 1":i32, "Line 1 & Line 2"=w414:i32, "Is Present"=w412:i32, "RC_AccessoryIsPresent"=w415:u32)
                        n195 = call "code translator.vi"("Error code"=w415) -> ("Error description"=→"AccessoryIsPresent":string)
                        n196 = call "code translator.vi"("Error code"=w414) -> ("Error description"=→"GetAccessory":string)
                        n197 = call "TRUEorFALSE.vi"("bool number"=w412) -> ("String"=→"Is Accessory ?":string)
                        n198 = local write "Set Accessory"(bool ?) -> ()
                      }
                    }
                  }
                }
              }
              frame #12 {
                # "Set Optical Params"
                n199 = case shown="True" "Set Params" {
                  tunnel: w425 -> [_ w430]
                  tunnel: "Focal tilt" -> [_ w429]
                  tunnel: "Angular deviation" -> [_ w428]
                  tunnel: "Focal length" -> [_ w427]
                  frame #0 {
                    n200 = local write "Initializing"(bool ?) -> ()
                  }
                  frame #1 {
                    n201 = stacked-sequence {
                      tunnel: w430 -> [_ w438]
                      tunnel: w429 -> [_ w435]
                      tunnel: w428 -> [_ w434]
                      tunnel: w427 -> [_ w433]
                      frame #0 {
                        n202 = local write "Initializing"(bool ?) -> ()
                      }
                      frame #1 {
                        n203 = call "atspectrograph_setOpticalParams.vi"("Focal Tilt"=w435, "Angular Deviation"=w434, "Focal Length"=w433, "Device No"=w438) -> ("RC_SetOpticalParameters"=w437:u32)
                        n204 = call "code translator.vi"("Error code"=w437) -> ("Error description"=→"Set Optical Parameters":string)
                        n205 = local write "Set Params"(bool ?) -> ()
                      }
                    }
                  }
                }
              }
            }
          }
        }
      }
    }
    frame #3 {
      n206 = call "shamrock_close.vi"() -> ("Close"=w440:u32)
      n207 = call "code translator.vi"("Error code"=w440) -> ("Error description"=→"Close":string)
    }
  }
